vi "SetHomePos.vi"(8 "error in (no error)":errorcluster caption="Fehler (Eingang, kein Fehler)", 11 "Moveo Eingang":refnum<class "Moveo.lvclass">) -> (0 "error out":errorcluster caption="Fehler (Ausgang)", 3 "Moveo Ausgang":refnum<class "Moveo.lvclass">)   [LabVIEW 2019, in "Moveo.lvclass"]
uses:
  Moveo.lvclass
  Moveo.lvclass/Moveo.ctl
  MoveoSerialClass/MoveoSerial.lvclass
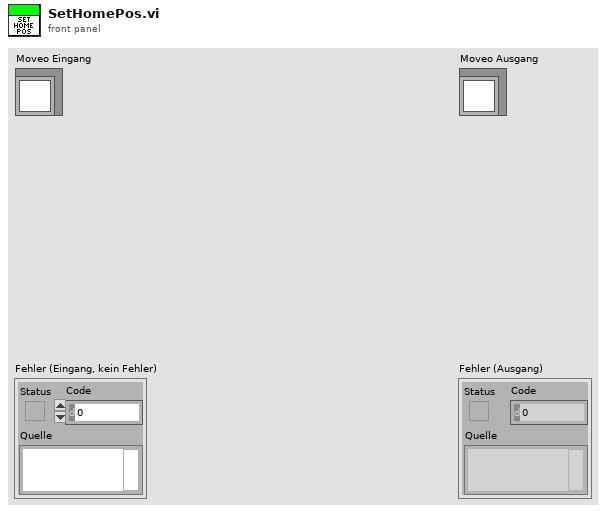
[diagram p1: front panel]
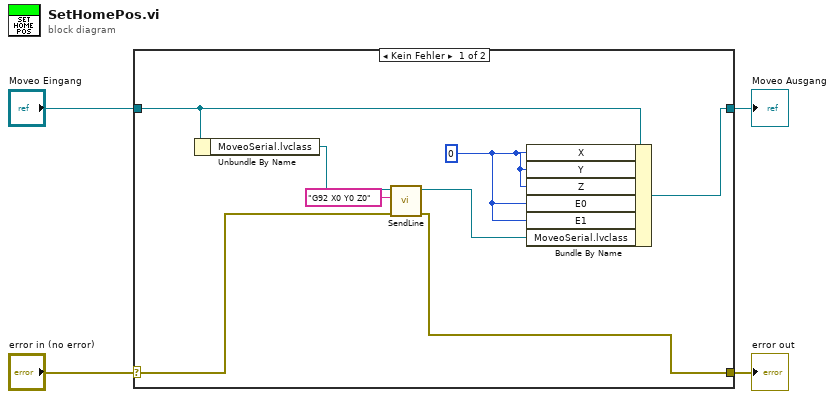
[diagram p0: block diagram]
diagram:
  n1 = case shown="Kein Fehler" "error in (no error)" {
    selector: "error in (no error)" -> [w6 w14]
    tunnel: [w5 w14] -> w3
    tunnel: [w9 w13] -> w1
    tunnel: "Moveo Eingang" -> [w10 w13]
    frame No Error {
      w8 = i16 0 ("X")
      n2 = Unbundle By Name(w10) -> ("MoveoSerial.lvclass"=w12:refnum<class "MoveoSerial.lvclass">)
      n3 = call-dynamic "SendLine.vi"("error in (no error)"=w6, "SendString"="G92 X0 Y0 Z0", "MoveoSerial Eingang"=w12) -> ("error out"=w5:errorcluster, "MoveoSerial Ausgang"=w7:refnum<class "MoveoSerial.lvclass">)  [unwired: 7 in]
      n4 = Bundle By Name(cluster=w10, "X"=w8, "Y"=w8, "Z"=w8, "E0"=w8, "E1"=w8, "MoveoSerial.lvclass"=w7) -> (w9:refnum<class "Moveo.lvclass">)
    }
    frame Error {
    }
  }
  "error out" <- w3
  "Moveo Ausgang" <- w1
